vi "demo_motor.vi"   [LabVIEW 2017]
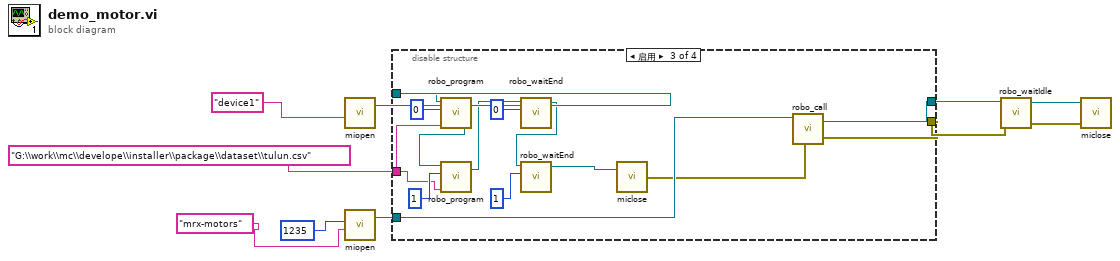
[diagram p0: block diagram]
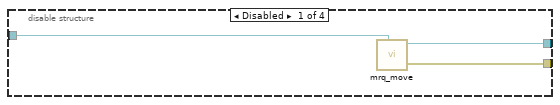
[diagram p2: hidden frame]
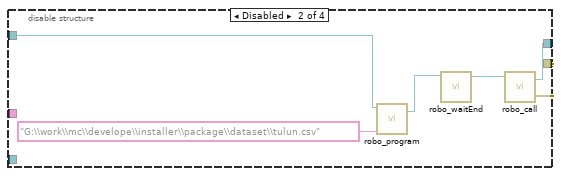
[diagram p3: hidden frame]
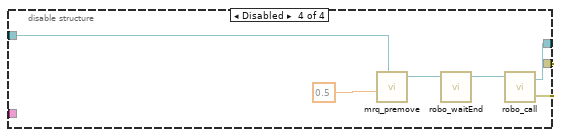
[diagram p4: hidden frame]
diagram:
  n1 = call "miopen.vi"("name"="device1") -> ("VISA资源名称输出"=w9:refnum<visa-resource-name>)  [unwired: 3 in, 1 out]
  n2 = call "miopen.vi"("name"="mrx-motors", "port"=u16 1235) -> ("VISA资源名称输出"=w1:refnum<visa-resource-name>)  [unwired: 2 in, 1 out]
  n3 = disable-structure shown="启用" {
    disable-tunnel: w9 -> [w13 w16 w31 w39]
    disable-tunnel: [w12 w18 w33 w36] -> w8
    disable-tunnel: [w11 w17 w32 w35] -> w7
    disable-tunnel: "G:\\work\\mc\\develope\\installer\\package\\dataset\\tulun.csv" ("file") -> [_ _ w25 _]
    disable-tunnel: w1 -> [_ _ w23 _]
    frame Disabled {
      n4 = call "mrq_move.vi"("VISA资源名称"=w13) -> ("VISA资源名称输出"=w12:refnum<visa-resource-name>, "错误输出"=w11:errorcluster)  [unwired: 6 in]
    }
    frame Disabled {
      n5 = call "robo_program.vi"("VISA资源名称"=w16, "file"="G:\\work\\mc\\develope\\installer\\package\\dataset\\tulun.csv") -> ("VISA资源名称输出"=w15:refnum<visa-resource-name>)  [unwired: 3 in, 1 out]
      n6 = call "robo_waitEnd.vi"("VISA资源名称"=w15) -> ("VISA资源名称输出"=w19:refnum<visa-resource-name>)  [unwired: 4 in, 2 out]
      n7 = call "robo_call.vi"("VISA资源名称"=w19) -> ("错误输出"=w17:errorcluster, "VISA资源名称输出"=w18:refnum<visa-resource-name>)  [unwired: 5 in]
    }
    frame Enabled {
      n8 = call "robo_program.vi"("VISA资源名称"=w31, "ax"=0, "file"=w25) -> ("VISA资源名称输出"=w30:refnum<visa-resource-name>)  [unwired: 2 in, 1 out]
      n9 = call "robo_program.vi"("VISA资源名称"=w30, "ax"=1, "file"=w25) -> ("VISA资源名称输出"=w28:refnum<visa-resource-name>)  [unwired: 2 in, 1 out]
      n10 = call "robo_waitEnd.vi"("VISA资源名称"=w28, "ax"=0) -> ("VISA资源名称输出"=w27:refnum<visa-resource-name>)  [unwired: 3 in, 2 out]
      n11 = call "robo_waitEnd.vi"("VISA资源名称"=w27, "ax"=1) -> ("VISA资源名称输出"=w24:refnum<visa-resource-name>)  [unwired: 3 in, 2 out]
      n12 = call "miclose.vi"("VISA资源名称"=w24) -> ("错误输出"=w22:errorcluster)  [unwired: 1 in]
      n13 = call "robo_call.vi"("错误输入（无错误）"=w22, "VISA资源名称"=w23) -> ("错误输出"=w32:errorcluster, "VISA资源名称输出"=w33:refnum<visa-resource-name>)  [unwired: 4 in]
    }
    frame Disabled {
      n14 = call "mrq_premove.vi"("VISA资源名称"=w39, "t"=sgl 0.5) -> ("VISA资源名称输出"=w38:refnum<visa-resource-name>)  [unwired: 5 in, 1 out]
      n15 = call "robo_waitEnd.vi"("VISA资源名称"=w38) -> ("VISA资源名称输出"=w37:refnum<visa-resource-name>)  [unwired: 4 in, 2 out]
      n16 = call "robo_call.vi"("VISA资源名称"=w37) -> ("错误输出"=w35:errorcluster, "VISA资源名称输出"=w36:refnum<visa-resource-name>)  [unwired: 5 in]
    }
  }
  n17 = call "robo_waitIdle.vi"("VISA资源名称"=w8, "错误输入（无错误）"=w7) -> ("VISA资源名称输出"=w6:refnum<visa-resource-name>, "错误输出"=w5:errorcluster)  [unwired: 3 in, 1 out]
  n18 = call "miclose.vi"("错误输入（无错误）"=w5, "VISA资源名称"=w6) -> ()  [unwired: 1 out]
